vi "Save_png_with_ROI.vi"() -> ()   [LabVIEW 2020]
uses:
  <vilib>/vision/NI_Vision_Development_Module.lvlib
panel:
  out "Image":T1(plugin-control)
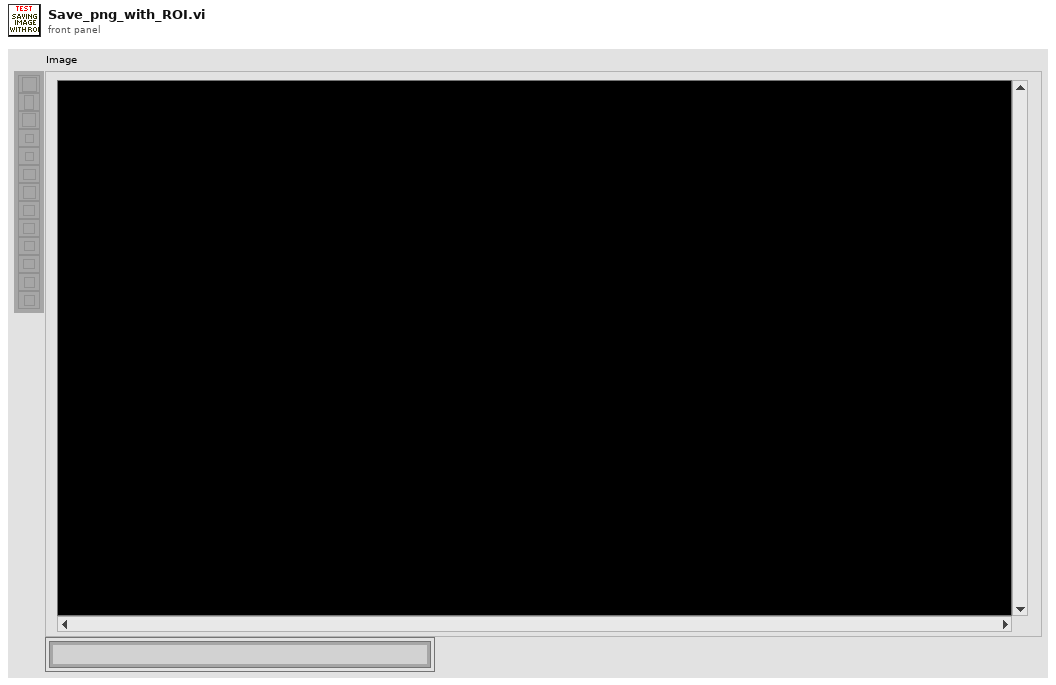
[diagram p1: front panel]
types:
  T1 = typedef "IMAQ Image.ctl" = refnum<image>
  T2 = typedef "Image Type" = u32
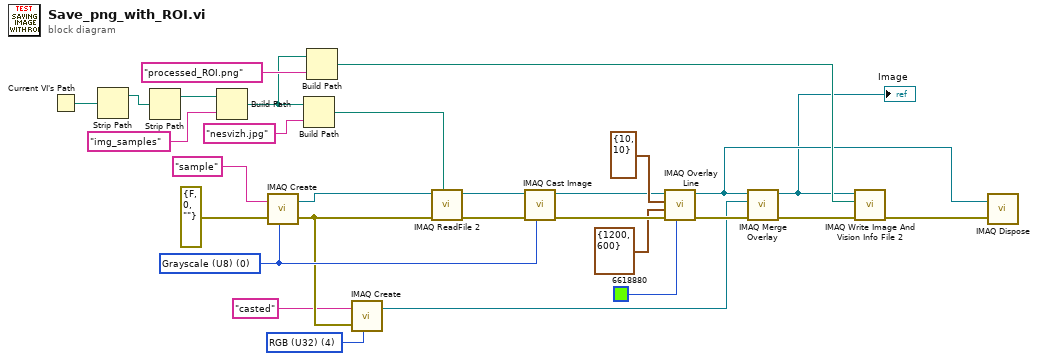
[diagram p0: block diagram]
diagram:
  w11 = T2 4 items=["Grayscale (U8)", "Grayscale (I16)", "Grayscale (SGL)", "Complex (CSG)", "RGB (U32)", "HSL (U32)", "RGB (U64)", "Grayscale (U16)"] ("Image Type")
  w21 = T2 0 items=["Grayscale (U8)", "Grayscale (I16)", "Grayscale (SGL)", "Complex (CSG)", "RGB (U32)", "HSL (U32)", "RGB (U64)", "Grayscale (U16)"] ("Image Type")
  n1 = Current VI's Path() -> (path=w26:path)
  n2 = Strip Path(path=w26) -> (stripped path=w4:path)  [unwired: 1 out]
  n3 = Strip Path(path=w4) -> (stripped path=w3:path)  [unwired: 1 out]
  n4 = Build Path(base path=w3, name or relative path="img_samples") -> (appended path=w1:path)
  n5 = call "IMAQ Create"("Image Name"="sample", "Image Type"=w21, "error in (no error)"=errorcluster {"status"=FALSE, "code"=0, "source"=""}) -> ("New Image"=w27:T1, "error out"=w13:errorcluster)  [unwired: 2 in]
  n6 = Build Path(base path=w1, name or relative path="nesvizh.jpg") -> (appended path=w24:path)
  n7 = Build Path(base path=w1, name or relative path="processed_ROI.png") -> (appended path=w14:path)
  n8 = call "IMAQ Create"("Image Name"="casted", "Image Type"=w11, "error in (no error)"=w13) -> ("New Image"=w9:T1)  [unwired: 2 in, 1 out]
  n9 = call "IMAQ ReadFile 2"("File Path"=w24, "error in (no error)"=w13, "Image"=w27) -> ("error out"=w23:errorcluster, "Image Out"=w22:T1)  [unwired: 4 in, 3 out]
  n10 = call "IMAQ Cast Image"("Image Type"=w21, "error in (no error)"=w23, "Image Src"=w22) -> ("error out"=w20:errorcluster, "Image Dst Out"=w16:T1)  [unwired: 7 in]
  n11 = call "IMAQ Overlay Line"("Color"=u32 6618880, "error in (no error)"=w20, "End Point"=cluster{"X":i32, "Y":i32} {"X"=1200, "Y"=600} ("Start Point"), "Start Point"=cluster{"X":i32, "Y":i32} {"X"=10, "Y"=10}, "Image"=w16) -> ("error out"=w10:errorcluster, "Image Out"=w6:T1)  [unwired: 5 in]
  n12 = call "IMAQ Merge Overlay"("error in (no error)"=w10, "Image Dst"=w9, "Image Src"=w6) -> ("error out"=w8:errorcluster, "Image Dst Out"=w5:T1)  [unwired: 7 in]
  "Image" <- w5
  n13 = call "IMAQ Write Image And Vision Info File 2"("error in (no error)"=w8, "File Path"=w14, "Image"=w5) -> ("error out"=w7:errorcluster)  [unwired: 7 in, 1 out]
  n14 = call "IMAQ Dispose"("Image"=w6, "error in (no error)"=w7) -> ()  [unwired: 4 in, 1 out]
